vi "Initialize.vi"(0 "Yokogawa WT1600 in":refnum<class "Yokogawa WT1600.lvclass">, 7 "Reset (T: Reset)":bool=TRUE, 9 "ID Query (T: Check)":bool=TRUE, 11 "error in (no error)":errorcluster) -> (4 "Yokogawa WT1600 out":refnum<class "Yokogawa WT1600.lvclass">, 6 "VISA resource name":refnum<visa-resource-name>, 15 "error out":errorcluster)   [LabVIEW 2013, in "Universal Power Meter.lvlib" / "Yokogawa WT1600.lvlib" / "Yokogawa WT1600.lvclass"]
uses:
  Yokogawa WT1600.lvclass
  Universal Power Meter class/Universal Power Meter.lvclass
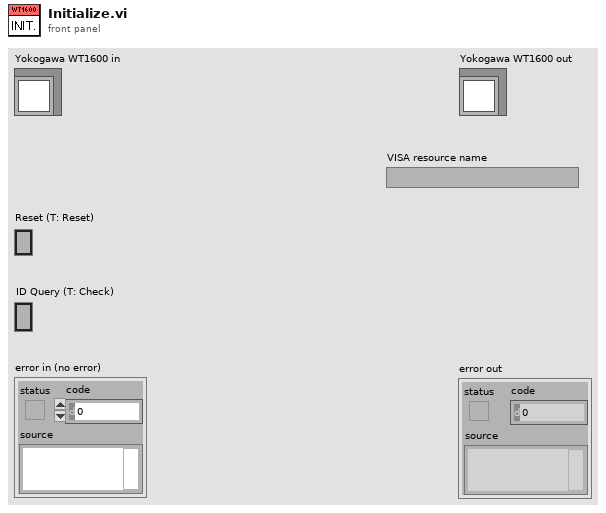
[diagram p1: front panel]
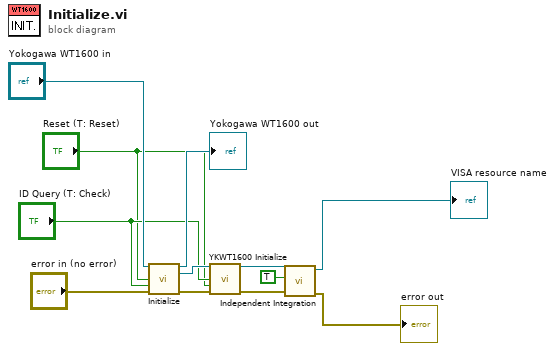
[diagram p0: block diagram]
diagram:
  n1 = call-parent "Initialize.vi"("Universal Power Meter in"="Yokogawa WT1600 in", "Reset (T: Reset)"="Reset (T: Reset)", "ID Query (T: Check)"="ID Query (T: Check)", "error in (no error)"="error in (no error)") -> ("Universal Power Meter out"=→"Yokogawa WT1600 out":refnum<class "Yokogawa WT1600.lvclass">, "VISA resource name"=w8:refnum<visa-resource-name>, "error out"=w9:errorcluster)  [unwired: 9 in]
  n2 = call <instrlib>:"YKWT1600 Initialize.vi"("VISA session (for class)"=w8, "ID Query (T: Check)"="ID Query (T: Check)", "Reset (T: Reset)"="Reset (T: Reset)", "error in (no error)"=w9) -> ("VISA session"=w5:refnum<visa-resource-name>, "error out"=w2:errorcluster)  [unwired: 10 in]
  n3 = call "Independent Integration.vi"("error in"=w2, "ON/OFF"=TRUE, "VISA resource name"=w5) -> ("error out"=→"error out":errorcluster, "VISA resource name out"=→"VISA resource name":refnum<visa-resource-name>)  [unwired: 7 in]
